vi "FFT - Spectrum Display Options.vi"(0 "Spectrum Display Options":T3, 1 "Spectral Function Type":T2, 2 "Acoustic Weighting":T1, 3 "Spectrum Mag IN":dbl[](array[numeric]), 4 "dF (Hz)":dbl=1.0, 5 "Unit IN":string) -> (17 "Spectrum Mag OUT":dbl[](array[numeric]), 18 "Unit OUT":string)   [LabVIEW 2022 SP3, in "GSwFormDSP.lvclass"]
uses:
  GSwFormDSP.lvclass
  Spectrum Display Options.ctl
  Spectral Function Type.ctl
  Acoustic Weighting.ctl
  Spectrum Mag Type.ctl
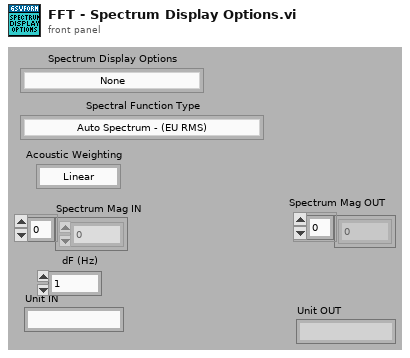
[diagram p1: front panel]
types:
  T1 = typedef "GSwFormDSP.lvclass/Acoustic Weighting.ctl" = enum16{"Linear", "A-weighting"}
  T2 = typedef "GSwFormDSP.lvclass/Spectral Function Type.ctl" = enum16{"Auto Spectrum - (EU RMS)", "Auto Spectrum - (EU Peak)", "Power Spectrum - (EU RMS²)", "Power Spectrum - (EU Peak²)", "Auto Spectrum Density - (EU RMS/rtHz)", "Auto Spectrum Density - (EU Peak/rtHz)", "Power Spectrum Density - (EU RMS²/Hz)", "Power Spectrum Density - (EU Peak²/Hz)"}
  T3 = typedef "GSwFormDSP.lvclass/Spectrum Display Options.ctl" = enum16{"None", "dB - NO reference value", "dB - Automatic reference value", "dB - Sound SPL (ref 20E-6 Pa)", "dB - Acceleration (ref 1E-6 m/s²)", "dB - Velocity (ref 1E-9 m/s)", "dB - Displacement (ref 1E-12 m)"}
  T4 = typedef "GSwFormDSP.lvclass/Spectrum Mag Type.ctl" = enum16{"dB", "EU", "EU²"}
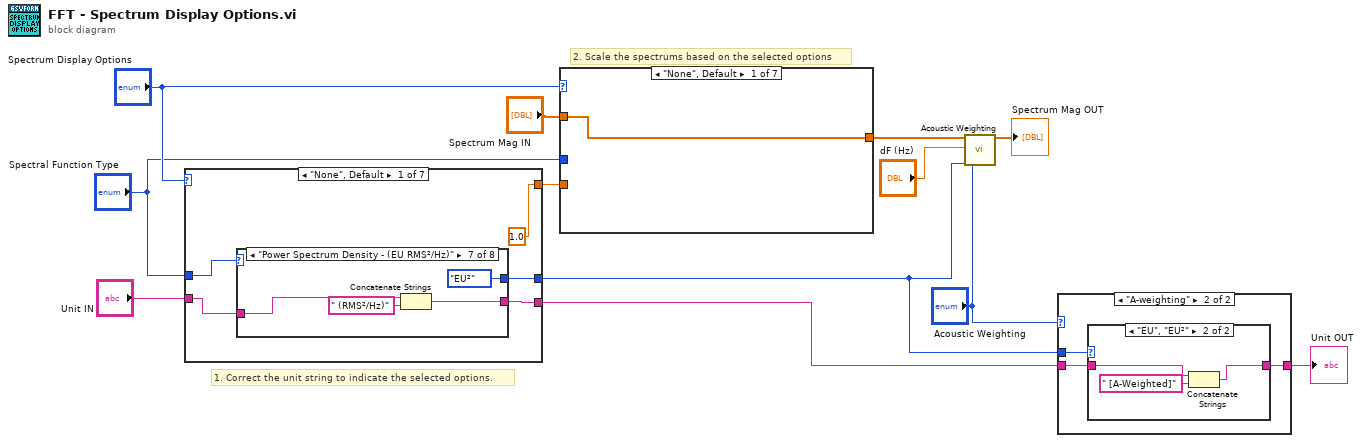
[diagram p0: block diagram]
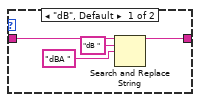
[diagram p3: hidden frame]
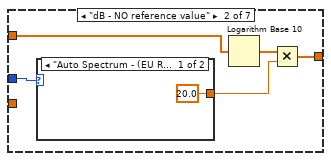
[diagram p4: hidden frame]
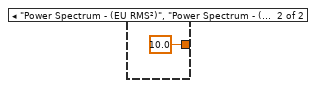
[diagram p5: hidden frame]
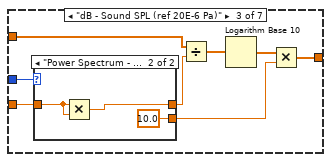
[diagram p6: hidden frame]
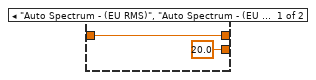
[diagram p7: hidden frame]
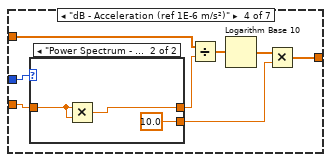
[diagram p8: hidden frame]
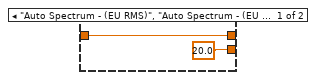
[diagram p9: hidden frame]
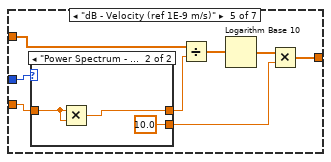
[diagram p10: hidden frame]
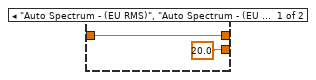
[diagram p11: hidden frame]
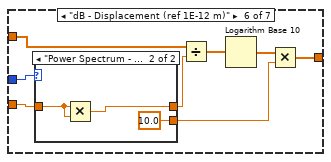
[diagram p12: hidden frame]
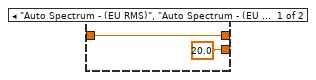
[diagram p13: hidden frame]
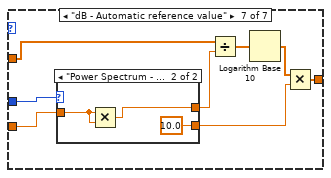
[diagram p14: hidden frame]
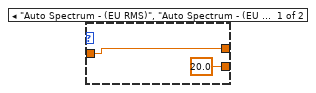
[diagram p15: hidden frame]
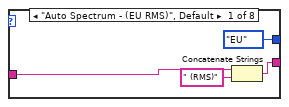
[diagram p16: hidden frame]
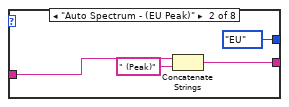
[diagram p17: hidden frame]
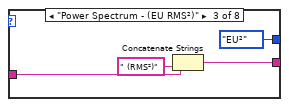
[diagram p18: hidden frame]
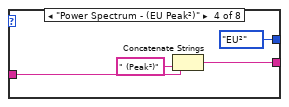
[diagram p19: hidden frame]
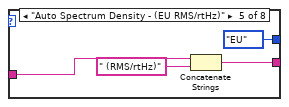
[diagram p20: hidden frame]
diagram:
  # "2. Scale the spectrums based on the selected options"
  # "1. Correct the unit string to indicate the selected options."
  n1 = case shown="\"None\", Default" "Spectrum Display Options" {
    tunnel: "Unit IN" -> [w17 w54 w71 w88 w105 w122 w138]
    tunnel: [w16 w53 w70 w87 w104 w121 w137] -> w3
    tunnel: "Spectral Function Type" -> [w15 w52 w69 w86 w103 w120 _]
    tunnel: [1.0 1.0 2e-05 1e-06 1e-09 1e-12 w136] -> w11
    tunnel: [w13 Spectrum_Mag_Type."dB" ("Spectrum Mag Type") Spectrum_Mag_Type."dB" ("Spectrum Mag Type") Spectrum_Mag_Type."dB" ("Spectrum Mag Type") Spectrum_Mag_Type."dB" ("Spectrum Mag Type") Spectrum_Mag_Type."dB" ("Spectrum Mag Type") Spectrum_Mag_Type."dB" ("Spectrum Mag Type")] -> w1
    frame "None", Default {
      n2 = case shown="\"Power Spectrum Density - (EU RMS²/Hz)\"" w15 {
        tunnel: w17 -> [w21 w25 w29 w33 w37 w41 w45 w49]
        tunnel: [w19 w23 w27 w31 w35 w39 w43 w47] -> w16
        tunnel: [Spectrum_Mag_Type."EU" ("Spectrum Mag Type") Spectrum_Mag_Type."EU" ("Spectrum Mag Type") Spectrum_Mag_Type."EU²" ("Spectrum Mag Type") Spectrum_Mag_Type."EU²" ("Spectrum Mag Type") Spectrum_Mag_Type."EU" ("Spectrum Mag Type") Spectrum_Mag_Type."EU" ("Spectrum Mag Type") Spectrum_Mag_Type."EU²" ("Spectrum Mag Type") Spectrum_Mag_Type."EU²" ("Spectrum Mag Type")] -> w13
        frame "Auto Spectrum - (EU RMS)", Default {
          n3 = Concatenate Strings(w21, " (RMS)" ("string")) -> (w19:string)
        }
        frame "Auto Spectrum - (EU Peak)" {
          n4 = Concatenate Strings(w25, " (Peak)" ("string")) -> (w23:string)
        }
        frame "Power Spectrum - (EU RMS²)" {
          n5 = Concatenate Strings(w29, " (RMS²)" ("string")) -> (w27:string)
        }
        frame "Power Spectrum - (EU Peak²)" {
          n6 = Concatenate Strings(w33, " (Peak²)" ("string")) -> (w31:string)
        }
        frame "Auto Spectrum Density - (EU RMS/rtHz)" {
          n7 = Concatenate Strings(w37, " (RMS/rtHz)" ("string")) -> (w35:string)
        }
        frame "Auto Spectrum Density - (EU Peak/rtHz)" {
          n8 = Concatenate Strings(w41, " (Peak/rtHz)" ("string")) -> (w39:string)
        }
        frame "Power Spectrum Density - (EU RMS²/Hz)" {
          n9 = Concatenate Strings(w45, " (RMS²/Hz)" ("string")) -> (w43:string)
        }
        frame "Power Spectrum Density - (EU Peak²/Hz)" {
          n10 = Concatenate Strings(w49, " (Peak²/Hz)" ("string")) -> (w47:string)
        }
      }
    }
    frame "dB - NO reference value" {
      n11 = case shown="\"Auto Spectrum - (EU RMS)\", \"Power Spectrum - (EU RMS²)\", Default" w52 {
        tunnel: w54 -> [w57 w60 w63 w66]
        tunnel: [w55 w58 w61 w64] -> w53
        frame "Auto Spectrum - (EU RMS)", "Power Spectrum - (EU RMS²)", Default {
          n12 = Concatenate Strings(w57, " (RMS [dB NoRef])" ("string")) -> (w55:string)
        }
        frame "Auto Spectrum - (EU Peak)", "Power Spectrum - (EU Peak²)" {
          n13 = Concatenate Strings(w60, " (Peak [dB NoRef])" ("string")) -> (w58:string)
        }
        frame "Auto Spectrum Density - (EU RMS/rtHz)", "Power Spectrum Density - (EU RMS²/Hz)" {
          n14 = Concatenate Strings(w63, " (RMS/Hz [dB NoRef])" ("string")) -> (w61:string)
        }
        frame "Auto Spectrum Density - (EU Peak/rtHz)", "Power Spectrum Density - (EU Peak²/Hz)" {
          n15 = Concatenate Strings(w66, " (Peak/Hz [dB NoRef])" ("string")) -> (w64:string)
        }
      }
    }
    frame "dB - Sound SPL (ref 20E-6 Pa)" {
      n16 = case shown="\"Auto Spectrum - (EU Peak)\", \"Power Spectrum - (EU Peak²)\"" w69 {
        tunnel: w71 -> [w74 w77 w80 w83]
        tunnel: [w72 w75 w78 w81] -> w70
        frame "Auto Spectrum - (EU RMS)", "Power Spectrum - (EU RMS²)", Default {
          n17 = Concatenate Strings(w74, " (RMS [dB 20µPa])" ("string")) -> (w72:string)
        }
        frame "Auto Spectrum - (EU Peak)", "Power Spectrum - (EU Peak²)" {
          n18 = Concatenate Strings(w77, " (Peak [dB 20µPa])" ("string")) -> (w75:string)
        }
        frame "Auto Spectrum Density - (EU RMS/rtHz)", "Power Spectrum Density - (EU RMS²/Hz)" {
          n19 = Concatenate Strings(w80, " (RMS/Hz [dB 20µPa])" ("string")) -> (w78:string)
        }
        frame "Auto Spectrum Density - (EU Peak/rtHz)", "Power Spectrum Density - (EU Peak²/Hz)" {
          n20 = Concatenate Strings(w83, " (Peak/Hz [dB 20µPa])" ("string")) -> (w81:string)
        }
      }
    }
    frame "dB - Acceleration (ref 1E-6 m/s²)" {
      n21 = case shown="\"Auto Spectrum - (EU Peak)\", \"Power Spectrum - (EU Peak²)\"" w86 {
        tunnel: w88 -> [w91 w94 w97 w100]
        tunnel: [w89 w92 w95 w98] -> w87
        frame "Auto Spectrum - (EU RMS)", "Power Spectrum - (EU RMS²)", Default {
          n22 = Concatenate Strings(w91, " (RMS [dB 1E-6 m/s²])" ("string")) -> (w89:string)
        }
        frame "Auto Spectrum - (EU Peak)", "Power Spectrum - (EU Peak²)" {
          n23 = Concatenate Strings(w94, " (Peak [dB 1E-6 m/s²])" ("string")) -> (w92:string)
        }
        frame "Auto Spectrum Density - (EU RMS/rtHz)", "Power Spectrum Density - (EU RMS²/Hz)" {
          n24 = Concatenate Strings(w97, " (RMS/Hz [dB 1E-6 m/s²])" ("string")) -> (w95:string)
        }
        frame "Auto Spectrum Density - (EU Peak/rtHz)", "Power Spectrum Density - (EU Peak²/Hz)" {
          n25 = Concatenate Strings(w100, " (Peak/Hz [dB 1E-6 m/s²])" ("string")) -> (w98:string)
        }
      }
    }
    frame "dB - Velocity (ref 1E-9 m/s)" {
      n26 = case shown="\"Auto Spectrum - (EU RMS)\", \"Power Spectrum - (EU RMS²)\", Default" w103 {
        tunnel: w105 -> [w108 w111 w114 w117]
        tunnel: [w106 w109 w112 w115] -> w104
        frame "Auto Spectrum - (EU RMS)", "Power Spectrum - (EU RMS²)", Default {
          n27 = Concatenate Strings(w108, " (RMS [dB 1E-9 m/s])" ("string")) -> (w106:string)
        }
        frame "Auto Spectrum - (EU Peak)", "Power Spectrum - (EU Peak²)" {
          n28 = Concatenate Strings(w111, " (Peak [dB 1E-9 m/s])" ("string")) -> (w109:string)
        }
        frame "Auto Spectrum Density - (EU RMS/rtHz)", "Power Spectrum Density - (EU RMS²/Hz)" {
          n29 = Concatenate Strings(w114, " (RMS/Hz [dB 1E-9 m/s])" ("string")) -> (w112:string)
        }
        frame "Auto Spectrum Density - (EU Peak/rtHz)", "Power Spectrum Density - (EU Peak²/Hz)" {
          n30 = Concatenate Strings(w117, " (Peak/Hz [dB 1E-9 m/s])" ("string")) -> (w115:string)
        }
      }
    }
    frame "dB - Displacement (ref 1E-12 m)" {
      n31 = case shown="\"Auto Spectrum - (EU RMS)\", \"Power Spectrum - (EU RMS²)\", Default" w120 {
        tunnel: w122 -> [w125 w128 w131 w134]
        tunnel: [w123 w126 w129 w132] -> w121
        frame "Auto Spectrum - (EU RMS)", "Power Spectrum - (EU RMS²)", Default {
          n32 = Concatenate Strings(w125, " (RMS [dB 1E-12 m])" ("string")) -> (w123:string)
        }
        frame "Auto Spectrum - (EU Peak)", "Power Spectrum - (EU Peak²)" {
          n33 = Concatenate Strings(w128, " (Peak [dB 1E-12 m])" ("string")) -> (w126:string)
        }
        frame "Auto Spectrum Density - (EU RMS/rtHz)", "Power Spectrum Density - (EU RMS²/Hz)" {
          n34 = Concatenate Strings(w131, " (RMS/Hz [dB 1E-12 m])" ("string")) -> (w129:string)
        }
        frame "Auto Spectrum Density - (EU Peak/rtHz)", "Power Spectrum Density - (EU Peak²/Hz)" {
          n35 = Concatenate Strings(w134, " (Peak/Hz [dB 1E-12 m])" ("string")) -> (w132:string)
        }
      }
    }
    frame "dB - Automatic reference value" {
      n36 = To Lower Case(string=w138) -> (all lower case string=w139:string)
      n37 = case shown="\"m/s^2\", \"m/s²\"" w139 {
        tunnel: [1.0 2e-05 1e-06 1e-09 1e-12] -> w136
        tunnel: w138 -> [w141 w146 w153 w158 w163]
        tunnel: [w143 w148 w152 w157 w162] -> w137
        frame "", Default {
          n38 = Concatenate Strings("dB [NoRef] (" ("string"), w141, ")" ("string")) -> (w143:string)
        }
        frame "pa" {
          n39 = Concatenate Strings(" dB [Ref 20µPa] (" ("string"), w146, ")" ("string")) -> (w148:string)
        }
        frame "m/s^2", "m/s²" {
          n40 = Concatenate Strings("dB [Ref 1E-6 m/s²] (" ("string"), w153, ")" ("string")) -> (w152:string)
        }
        frame "m/s" {
          n41 = Concatenate Strings("dB [Ref 1E-9 m/s] (" ("string"), w158, ")" ("string")) -> (w157:string)
        }
        frame "m" {
          n42 = Concatenate Strings("dB [Ref 1E-12 m] (" ("string"), w163, ")" ("string")) -> (w162:string)
        }
      }
    }
  }
  n43 = case shown="\"None\", Default" "Spectrum Display Options" {
    tunnel: [w165 w166 w179 w191 w204 w217 w230] -> w7
    tunnel: "Spectrum Mag IN" -> [w165 w170 w178 w190 w203 w216 w229]
    tunnel: "Spectral Function Type" -> [_ w167 w175 w187 w200 w213 w227]
    tunnel: w11 -> [_ _ w174 w186 w199 w212 w225]
    frame "None", Default {
    }
    frame "dB - NO reference value" {
      n44 = case shown="\"Auto Spectrum - (EU RMS)\", \"Auto Spectrum - (EU Peak)\", \"Auto Spectrum Density - (EU RMS/rtHz)\", \"Auto Spectrum Density - (EU Peak/rtHz)\", Default" w167 {
        tunnel: [20.0 10.0] -> w168
        frame "Auto Spectrum - (EU RMS)", "Auto Spectrum - (EU Peak)", "Auto Spectrum Density - (EU RMS/rtHz)", "Auto Spectrum Density - (EU Peak/rtHz)", Default {
        }
        frame "Power Spectrum - (EU RMS²)", "Power Spectrum - (EU Peak²)", "Power Spectrum Density - (EU RMS²/Hz)", "Power Spectrum Density - (EU Peak²/Hz)" {
        }
      }
      n45 = Logarithm Base 10(1:w170) -> (0:w169:dbl[])
      n46 = Multiply(x=w169, y=w168) -> (x*y=w166:dbl[])
    }
    frame "dB - Sound SPL (ref 20E-6 Pa)" {
      n47 = case shown="\"Power Spectrum - (EU RMS²)\", \"Power Spectrum - (EU Peak²)\", \"Power Spectrum Density - (EU RMS²/Hz)\", \"Power Spectrum Density - (EU Peak²/Hz)\"" w175 {
        tunnel: [20.0 10.0] -> w173
        tunnel: [w181 w183] -> w176
        tunnel: w174 -> [w181 w184]
        frame "Auto Spectrum - (EU RMS)", "Auto Spectrum - (EU Peak)", "Auto Spectrum Density - (EU RMS/rtHz)", "Auto Spectrum Density - (EU Peak/rtHz)", Default {
        }
        frame "Power Spectrum - (EU RMS²)", "Power Spectrum - (EU Peak²)", "Power Spectrum Density - (EU RMS²/Hz)", "Power Spectrum Density - (EU Peak²/Hz)" {
          n48 = Multiply(x=w184, y=w184) -> (x*y=w183:dbl)
        }
      }
      n49 = Divide(x=w178, y=w176) -> (x/y=w177:dbl[])
      n50 = Logarithm Base 10(1:w177) -> (0:w180:dbl[])
      n51 = Multiply(x=w180, y=w173) -> (x*y=w179:dbl[])
    }
    frame "dB - Acceleration (ref 1E-6 m/s²)" {
      n52 = case shown="\"Power Spectrum - (EU RMS²)\", \"Power Spectrum - (EU Peak²)\", \"Power Spectrum Density - (EU RMS²/Hz)\", \"Power Spectrum Density - (EU Peak²/Hz)\"" w187 {
        tunnel: [20.0 10.0] -> w192
        tunnel: [w194 w196] -> w188
        tunnel: w186 -> [w194 w197]
        frame "Auto Spectrum - (EU RMS)", "Auto Spectrum - (EU Peak)", "Auto Spectrum Density - (EU RMS/rtHz)", "Auto Spectrum Density - (EU Peak/rtHz)", Default {
        }
        frame "Power Spectrum - (EU RMS²)", "Power Spectrum - (EU Peak²)", "Power Spectrum Density - (EU RMS²/Hz)", "Power Spectrum Density - (EU Peak²/Hz)" {
          n53 = Multiply(x=w197, y=w197) -> (x*y=w196:dbl)
        }
      }
      n54 = Divide(x=w190, y=w188) -> (x/y=w189:dbl[])
      n55 = Logarithm Base 10(1:w189) -> (0:w193:dbl[])
      n56 = Multiply(x=w193, y=w192) -> (x*y=w191:dbl[])
    }
    frame "dB - Velocity (ref 1E-9 m/s)" {
      n57 = case shown="\"Power Spectrum - (EU RMS²)\", \"Power Spectrum - (EU Peak²)\", \"Power Spectrum Density - (EU RMS²/Hz)\", \"Power Spectrum Density - (EU Peak²/Hz)\"" w200 {
        tunnel: [20.0 10.0] -> w205
        tunnel: [w207 w209] -> w201
        tunnel: w199 -> [w207 w210]
        frame "Auto Spectrum - (EU RMS)", "Auto Spectrum - (EU Peak)", "Auto Spectrum Density - (EU RMS/rtHz)", "Auto Spectrum Density - (EU Peak/rtHz)", Default {
        }
        frame "Power Spectrum - (EU RMS²)", "Power Spectrum - (EU Peak²)", "Power Spectrum Density - (EU RMS²/Hz)", "Power Spectrum Density - (EU Peak²/Hz)" {
          n58 = Multiply(x=w210, y=w210) -> (x*y=w209:dbl)
        }
      }
      n59 = Divide(x=w203, y=w201) -> (x/y=w202:dbl[])
      n60 = Logarithm Base 10(1:w202) -> (0:w206:dbl[])
      n61 = Multiply(x=w206, y=w205) -> (x*y=w204:dbl[])
    }
    frame "dB - Displacement (ref 1E-12 m)" {
      n62 = case shown="\"Power Spectrum - (EU RMS²)\", \"Power Spectrum - (EU Peak²)\", \"Power Spectrum Density - (EU RMS²/Hz)\", \"Power Spectrum Density - (EU Peak²/Hz)\"" w213 {
        tunnel: [20.0 10.0] -> w218
        tunnel: [w220 w222] -> w214
        tunnel: w212 -> [w220 w223]
        frame "Auto Spectrum - (EU RMS)", "Auto Spectrum - (EU Peak)", "Auto Spectrum Density - (EU RMS/rtHz)", "Auto Spectrum Density - (EU Peak/rtHz)", Default {
        }
        frame "Power Spectrum - (EU RMS²)", "Power Spectrum - (EU Peak²)", "Power Spectrum Density - (EU RMS²/Hz)", "Power Spectrum Density - (EU Peak²/Hz)" {
          n63 = Multiply(x=w223, y=w223) -> (x*y=w222:dbl)
        }
      }
      n64 = Divide(x=w216, y=w214) -> (x/y=w215:dbl[])
      n65 = Logarithm Base 10(1:w215) -> (0:w219:dbl[])
      n66 = Multiply(x=w219, y=w218) -> (x*y=w217:dbl[])
    }
    frame "dB - Automatic reference value" {
      n67 = case shown="\"Power Spectrum - (EU RMS²)\", \"Power Spectrum - (EU Peak²)\", \"Power Spectrum Density - (EU RMS²/Hz)\", \"Power Spectrum Density - (EU Peak²/Hz)\"" w227 {
        tunnel: [20.0 10.0] -> w231
        tunnel: w225 -> [w233 w236]
        tunnel: [w233 w235] -> w226
        frame "Auto Spectrum - (EU RMS)", "Auto Spectrum - (EU Peak)", "Auto Spectrum Density - (EU RMS/rtHz)", "Auto Spectrum Density - (EU Peak/rtHz)", Default {
        }
        frame "Power Spectrum - (EU RMS²)", "Power Spectrum - (EU Peak²)", "Power Spectrum Density - (EU RMS²/Hz)", "Power Spectrum Density - (EU Peak²/Hz)" {
          n68 = Multiply(x=w236, y=w236) -> (x*y=w235:dbl)
        }
      }
      n69 = Divide(x=w229, y=w226) -> (x/y=w228:dbl[])
      n70 = Logarithm Base 10(1:w228) -> (0:w232:dbl[])
      n71 = Multiply(x=w232, y=w231) -> (x*y=w230:dbl[])
    }
  }
  n72 = call "Acoustic Weighting.vi"("Spectrum"=w7, "dF (Hz)"="dF (Hz)", "Spectrum Mag Type"=w1, "Acoustic Weighting"="Acoustic Weighting") -> ("Weighted Spectrum"=→"Spectrum Mag OUT":dbl[])  [unwired: 15 in]
  n73 = case shown="\"A-weighting\"" "Acoustic Weighting" {
    tunnel: [w238 w240] -> w4
    tunnel: w3 -> [w238 w241]
    tunnel: w1 -> [_ w239]
    frame "Linear", Default {
    }
    frame "A-weighting" {
      n74 = case shown="\"EU\", \"EU²\"" w239 {
        tunnel: w241 -> [w245 w247]
        tunnel: [w244 w246] -> w240
        frame "dB", Default {
          n75 = Search and Replace String(input string=w245, search string="dB ", replace string="dBA " ("search string")) -> (result string=w244:string)  [unwired: 5 in, 3 out]
        }
        frame "EU", "EU²" {
          n76 = Concatenate Strings(w247, " [A-Weighted]" ("string")) -> (w246:string)
        }
      }
    }
  }
  "Unit OUT" <- w4
